vi "ArrayView1005.vi"   [LabVIEW 2013]
uses:
  <vilib>/Heliosphere Research LLC/Advanced Plotting Toolkit/api_plotting/ArrayViewProperties.ctl
  <vilib>/Heliosphere Research LLC/Advanced Plotting Toolkit/properties/Colormap.ctl
  <vilib>/Heliosphere Research LLC/Advanced Plotting Toolkit/properties/Colormap_Map.ctl
  <vilib>/Heliosphere Research LLC/Advanced Plotting Toolkit/properties/Colormap_Scaling.ctl
  <vilib>/Heliosphere Research LLC/Advanced Plotting Toolkit/properties/Display.ctl
  <vilib>/Heliosphere Research LLC/Advanced Plotting Toolkit/Advanced Plotting Toolkit.lvlib
types:
  T1 = typedef "Advanced Plotting Toolkit.lvlib/ArrayViewProperties.ctl" = cluster{"Colormap":T2, "Display":T5}
  T2 = typedef "Advanced Plotting Toolkit.lvlib/Colormap.ctl" = cluster{"Map":T3, "Value Min":dbl, "Value Max":dbl, "Scaling":T4, "Reverse":bool}
  T3 = typedef "Advanced Plotting Toolkit.lvlib/Colormap_Map.ctl" = enum16{"Automatic", "Rainbow", "Hot and Cold", "White-Black", "White-Blue", "White-Green", "White-Red", "Fire", "Water", "Earth", "Air", "Pastel", "Banded", "Stepped"}
  T4 = typedef "Advanced Plotting Toolkit.lvlib/Colormap_Scaling.ctl" = enum16{"Default", "Linear", "Log10"}
  T5 = typedef "Advanced Plotting Toolkit.lvlib/Display.ctl" = cluster{"Alpha":dbl, "Z Order":dbl}
  T6 = typedef "Advanced Plotting Toolkit.lvlib/PlotID.ctl" = i32
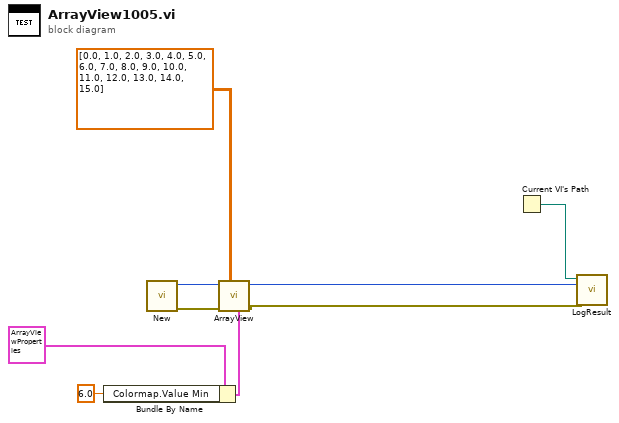
[diagram p0: block diagram]
diagram:
  n1 = Bundle By Name(cluster=T1 {"Colormap"={"Map"=enum."Automatic", "Value Min"=nan, "Value Max"=nan, "Scaling"=enum."Default", "Reverse"=FALSE}, "Display"={"Alpha"=nan, "Z Order"=nan}} ("Array View Properties"), "Colormap.Value Min"=6.0) -> (w2:T1)
  n2 = call <vilib>:"New.vi"() -> ("error out"=w5:errorcluster, "Plot ID"=w6:T6)  [unwired: 10 in]
  n3 = call <vilib>:"ArrayView.vi"("Properties"=w2, "Data"=dbl[][] [[0.0, 1.0, 2.0, 3.0], [4.0, 5.0, 6.0, 7.0], [8.0, 9.0, 10.0, 11.0], [12.0, 13.0, 14.0, 15.0]], "error in (no error)"=w5, "Plot ID"=w6) -> ("error out"=w4:errorcluster, "Plot ID Out"=w7:T6)  [unwired: 6 in]
  n4 = Current VI's Path() -> (path=w9:path)
  n5 = call "LogResult.vi"("Test Result"=w4, "Test Artifact"=w7, "VI Path"=w9) -> ()  [unwired: 9 in]
